vi "Write Buses.vi"(8 "error in (no error)":errorcluster, 10 "Buses":refnum<class "Bus_Access.lvclass">[](array[class]), 11 "Remap Bus in":refnum<class "Alias Bus.lvclass">) -> (0 "error out":errorcluster, 3 "Remap Bus out":refnum<class "Alias Bus.lvclass">)   [LabVIEW 2021, in "Alias Bus.lvclass"]
uses:
  Alias Bus.lvclass
  Omni-Bus/Bus Access/Bus_Access.lvclass
  Alias Bus.lvclass/Alias Bus.ctl
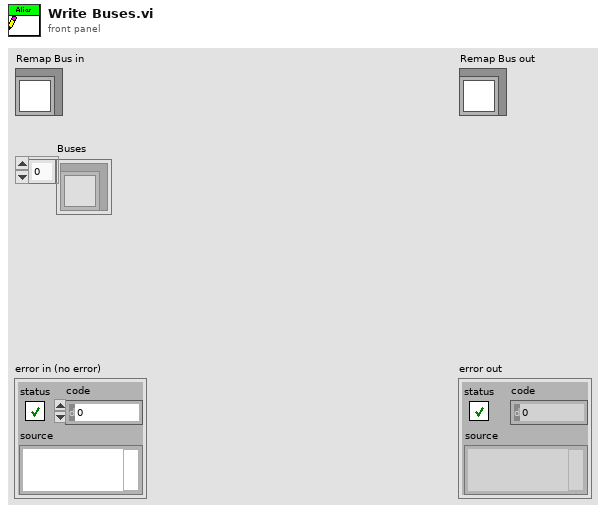
[diagram p1: front panel]
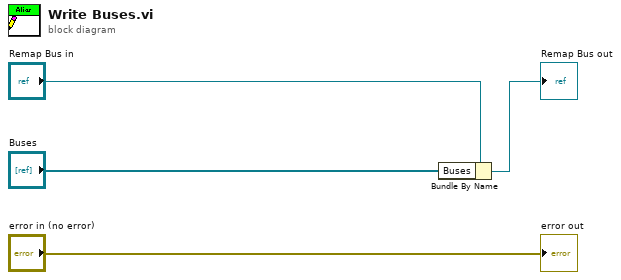
[diagram p0: block diagram]
diagram:
  n1 = Bundle By Name(cluster="Remap Bus in", "Buses"="Buses") -> (→"Remap Bus out":refnum<class "Alias Bus.lvclass">)
  "error out" <- "error in (no error)"
